vi "process_layer_parameter_strings_to_strict_type.vi"(8 "error in (no error)":errorcluster, 10 "Process layer parameters (strings)":T2) -> (0 "error out":errorcluster, 2 "Process layer parameters":T1 {"Final Thick (kA)" format="%_6g"})   [LabVIEW 2018]
uses:
  process_layer_parameters_strings.ctl
  process_layer_parameters.ctl
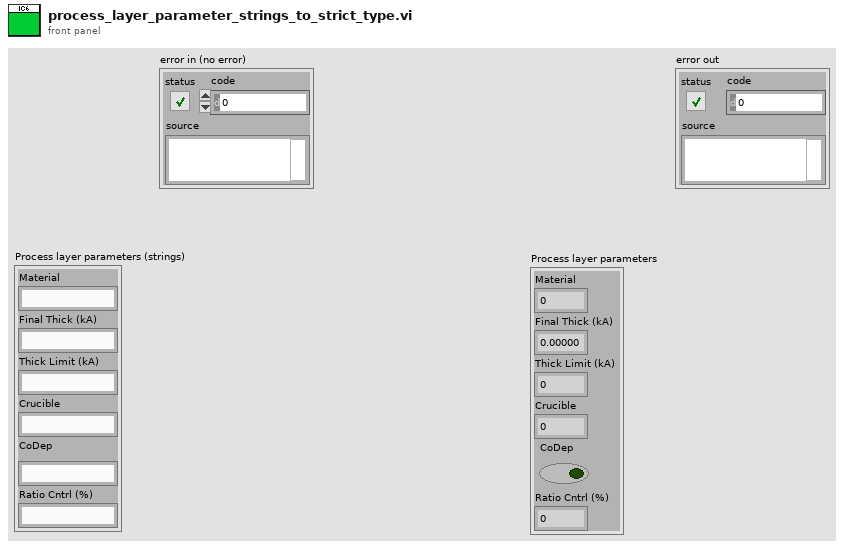
[diagram p1: front panel]
types:
  T1 = typedef "process_layer_parameters.ctl" = cluster{"Material":u8, "Final Thick (kA)":sgl, "Thick Limit (kA)":sgl, "Crucible":u8, "CoDep":bool, "Ratio Cntrl (%)":sgl}
  T2 = typedef "process_layer_parameters_strings.ctl" = cluster{"Material":string, "Final Thick (kA)":string, "Thick Limit (kA)":string, "Crucible":string, "CoDep":string, "Ratio Cntrl (%)":string}
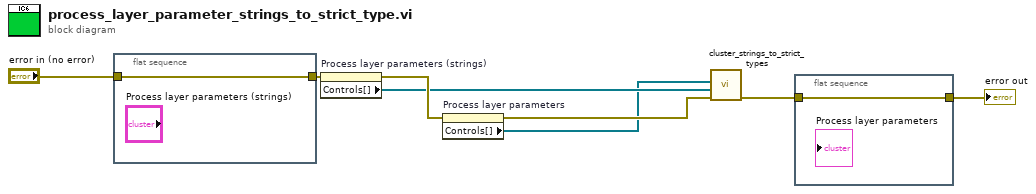
[diagram p0: block diagram]
diagram:
  n1 = flat-sequence {
    tunnel: "error in (no error)" -> [w9]
    tunnel: [w9] -> w7
    frame #0 {
    }
  }
  n2 = property on="Process layer parameters (strings)" class="Clust (strict)"(error in=w7) -> (error out=w5:errorcluster, "Controls[]"=w4:refnum<vi>[])  [unwired: 1 in, 1 out]
  n3 = property on="Process layer parameters" class="Clust (strict)"(error in=w5) -> (error out=w3:errorcluster, "Controls[]"=w2:refnum<vi>[])  [unwired: 1 in, 1 out]
  n4 = call "cluster_strings_to_strict_types.vi"("error in (no error)"=w3, "Controls[] (strings)"=w4, "Controls[]"=w2) -> ("error out"=w1:errorcluster)  [unwired: 8 in]
  n5 = flat-sequence {
    tunnel: w1 -> [w10]
    tunnel: [w10] -> w6
    frame #0 {
    }
  }
  "error out" <- w6
